vi "rdb_json_decode_constant.vi"(8 "error in (no error)":errorcluster, 9 "offset (0)":i32, 11 "json":string) -> (0 "error out":errorcluster, 1 "offset past match":i32, 2 "value":variant, 3 "type":T1)   [LabVIEW 2017]
uses:
  rdb_json_type.ctl
  <vilib>/Utility/error.llb/Error Cluster From Error Code.vi
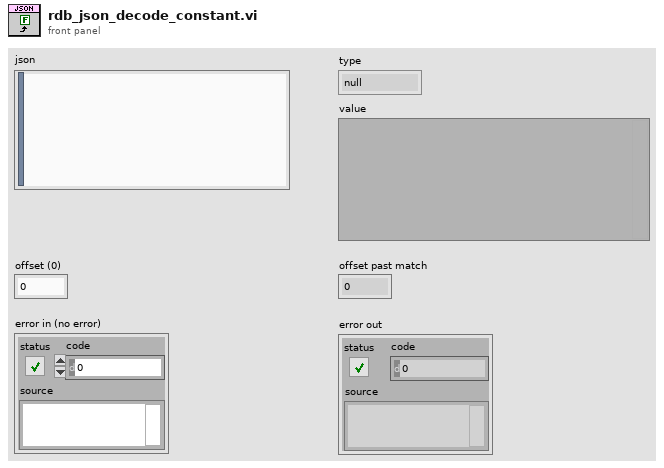
[diagram p1: front panel]
types:
  T1 = typedef "rdb_json_type.ctl" = enum8{"null", "bool", "int", "uint", "float", "string", "array", "object", "invalid"}
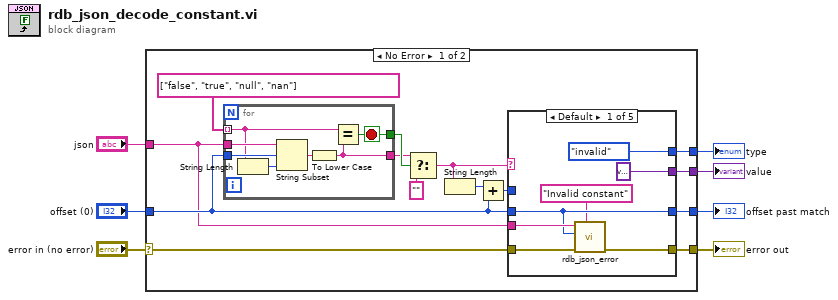
[diagram p0: block diagram]
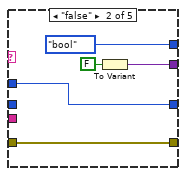
[diagram p2: hidden frame]
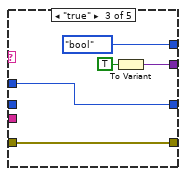
[diagram p3: hidden frame]
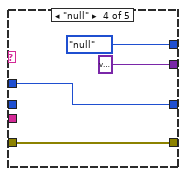
[diagram p4: hidden frame]
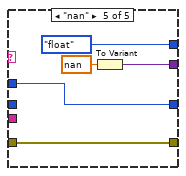
[diagram p5: hidden frame]
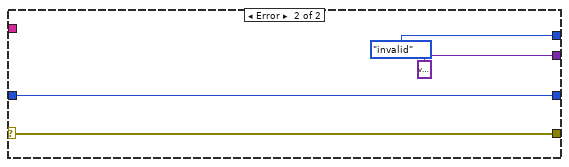
[diagram p6: hidden frame]
diagram:
  n1 = case shown="No Error" "error in (no error)" {
    selector: "error in (no error)" -> [w20 w58]
    tunnel: "json" -> [w8 _]
    tunnel: [w21 w58] -> w6
    tunnel: "offset (0)" -> [w10 w57]
    tunnel: [w15 w57] -> w3
    tunnel: [w14 rdb_json_type."invalid" ("type")] -> w2
    tunnel: [w13 variant ("Variant")] -> w1
    frame No Error {
      n2 = for {
        tunnel: w8 -> [w54]
        tunnel: w10 -> [w52]
        tunnel: string[] ["false", "true", "null", "nan"] -> [w51] mode=indexing
        tunnel: [w49] -> w17
        tunnel: [w48] -> w18
        stop <- w48 stop-if-true
        n3 = String Length(string=w51) -> (length=w53:i32)
        n4 = String Subset(string=w54, offset (0)=w52, length (rest)=w53) -> (substring=w50:string)
        n5 = To Lower Case(string=w50) -> (all lower case string=w49:string)
        n6 = Equal?(x=w51, y=w49) -> (x = y?=w48:bool)
      }
      n7 = Select(t=w17, s=w18, f="") -> (s? t:f=w12:string)
      n8 = String Length(string=w12) -> (length=w11:i32)
      n9 = Add(x=w11, y=w10) -> (x+y=w9:i32)
      n10 = case shown="Default" w12 {
        tunnel: w10 -> [w24 _ _ _ _]
        tunnel: [w23 w33 w38 w42 w47] -> w21
        tunnel: w20 -> [w26 w33 w38 w42 w47]
        tunnel: [w24 w29 w34 w39 w43] -> w15
        tunnel: [rdb_json_type."invalid" ("type") rdb_json_type."bool" ("type") rdb_json_type."bool" ("type") rdb_json_type."null" ("type") rdb_json_type."float" ("type")] -> w14
        tunnel: [variant ("Variant") w31 w36 variant ("value") w44] -> w13
        tunnel: w9 -> [_ w29 w34 w39 w43]
        tunnel: w8 -> [w25 _ _ _ _]
        frame Default {
          n11 = call "rdb_json_error.vi"("message"="Invalid constant" ("error message (\"\")"), "error in (no error)"=w26, "offset (0)"=w24, "json"=w25) -> ("error out"=w23:errorcluster)  [unwired: 7 in]
        }
        frame "false" {
          n12 = To Variant(anything=FALSE) -> (Variant=w31:variant)
        }
        frame "true" {
          n13 = To Variant(anything=TRUE) -> (Variant=w36:variant)
        }
        frame "null" {
        }
        frame "nan" {
          n14 = To Variant(anything=nan) -> (Variant=w44:variant)
        }
      }
    }
    frame Error {
    }
  }
  "error out" <- w6
  "offset past match" <- w3
  "type" <- w2
  "value" <- w1
